vi "identify line.vi"(3 "index":u8=1, 4 "points":cluster{"x":i16, "y":i16}[](array[cluster]), 5 "location":cluster{"x":i16, "y":i16}, 6 "8-bit pixmap":u8[][](array[numeric])) -> (0 "relative to location":cluster{"direction":dbl, "distance":dbl}, 2 "direction":dbl)   [LabVIEW 2009]
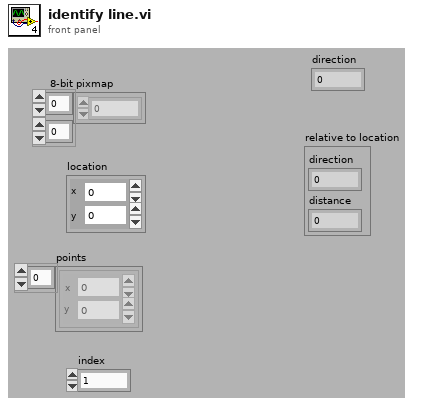
[diagram p1: front panel]
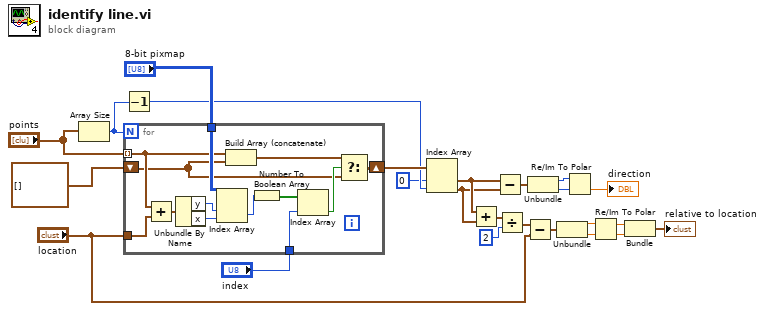
[diagram p0: block diagram]
diagram:
  n1 = Array Size(array="points") -> (size(s)=w16:i32)
  n2 = Decrement(x=w16) -> (x-1=w17:i32)
  n3 = for {
    N: w16 -> [_]
    tunnel: "points" -> [w27] mode=indexing
    tunnel: "8-bit pixmap" -> [w37]
    shift-right: [w30] -> w18
    shift-left: cluster{"x":i16, "y":i16}[] [] ("points along perimeter") -> [w26]
    tunnel: "index" -> [w28]
    tunnel: "location" -> [w25]
    n4 = Add(x=w27, y=w25) -> (x+y=w33:cluster{"x":i16, "y":i16})
    n5 = Unbundle By Name(w33) -> ("y"=w31:i16, "x"=w32:i16)
    n6 = Index Array(array=w37, index (row)=w31, index (col)=w32) -> (element=w34:u8)
    n7 = Build Array (concatenate)(w27, w26) -> (w35:cluster{"x":i16, "y":i16}[])
    n8 = Number To Boolean Array(number=w34) -> (Boolean array=w36:bool[])
    n9 = Index Array(array=w36, index=w28) -> (element=w29:bool)
    n10 = Select(t=w35, s=w29, f=w26) -> (s? t:f=w30:cluster{"x":i16, "y":i16}[])
  }
  n11 = Index Array(array=w18, index #1=0 ("index"), index #2=w17) -> (element #1=w12:cluster{"x":i16, "y":i16}, element #2=w11:cluster{"x":i16, "y":i16})
  n12 = Add(x=w12, y=w11) -> (x+y=w10:cluster{"x":i16, "y":i16})
  n13 = Subtract(x=w12, y=w11) -> (x-y=w21:cluster{"x":i16, "y":i16})
  n14 = Divide(x=w10, y=2) -> (x/y=w8:cluster{"x":dbl, "y":dbl})
  n15 = Subtract(x=w8, y="location") -> (x-y=w6:cluster{"x":dbl, "y":dbl})
  n16 = Unbundle(w21) -> ("x"=w20:i16, "y"=w19:i16)
  n17 = Unbundle(w6) -> ("x"=w5:dbl, "y"=w4:dbl)
  n18 = Re/Im To Polar(2:w19, 3:w20) -> (0:→"direction":dbl)  [unwired: 1 out]
  n19 = Re/Im To Polar(2:w4, 3:w5) -> (0:w3:dbl, 1:w2:dbl)
  n20 = Bundle(w2, w3) -> (→"relative to location":cluster{dbl, dbl})  [unwired: 1 in]
